vi "FieldByStepRotationForYakunin.vi"() -> ()   [LabVIEW 2019]
panel:
  in  "Rotator position Min":dbl
  in  "Rotator Position Max":dbl
  out "Direct Field Step:\nCurrent Value":dbl=0.1
  in  "Field Step Tab Control":enum32{"Direct Field", "Reciprocal Field"}(tab)
  in  "Direct Field Step (T)":dbl=0.1
  in  "DFS: Direct Field Step (T)":dbl=0.1
  in  "RFS: Reciprocal Field Step (1/T)":dbl=0.01
  in  "Threshold (T)":dbl=5.0
  in  "Calculate Setpoint":bool
  out "Power Supply State":string
  in  "Power Supply State":T1(ring)
  in  "Field:Rate [T/min]":dbl=0.2 min=0.0 max=0.6
  in  "Field:Final Setpoint":dbl min=-18.0 max=18.0
  out "Field: Current Value":dbl
  in  "stop":bool
  out "Field Runs":bool
  out "Field: Current Setpoint":dbl format="%.5f"
  out "Measurement Runs":bool
  in  "Steady Field":bool=TRUE
  # "Direct Field Step (DFS) will not be\nchanged below Threshold; while above: DFS=RFS*Field^2"
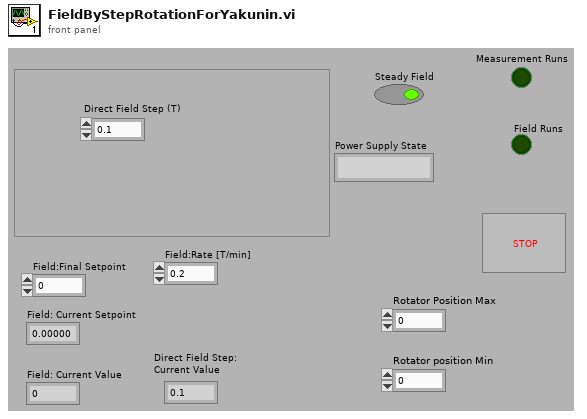
[diagram p1: front panel]
types:
  T1 = enum16{"No Response", "Ramping to programmed field ", "Holding at programmed field", "Paused", "Ramp Manual Up", "Ramp Manual Down", "Ramping to Zero", "QUENCH", "Heating Persistance Switch", "At Zero Current"}
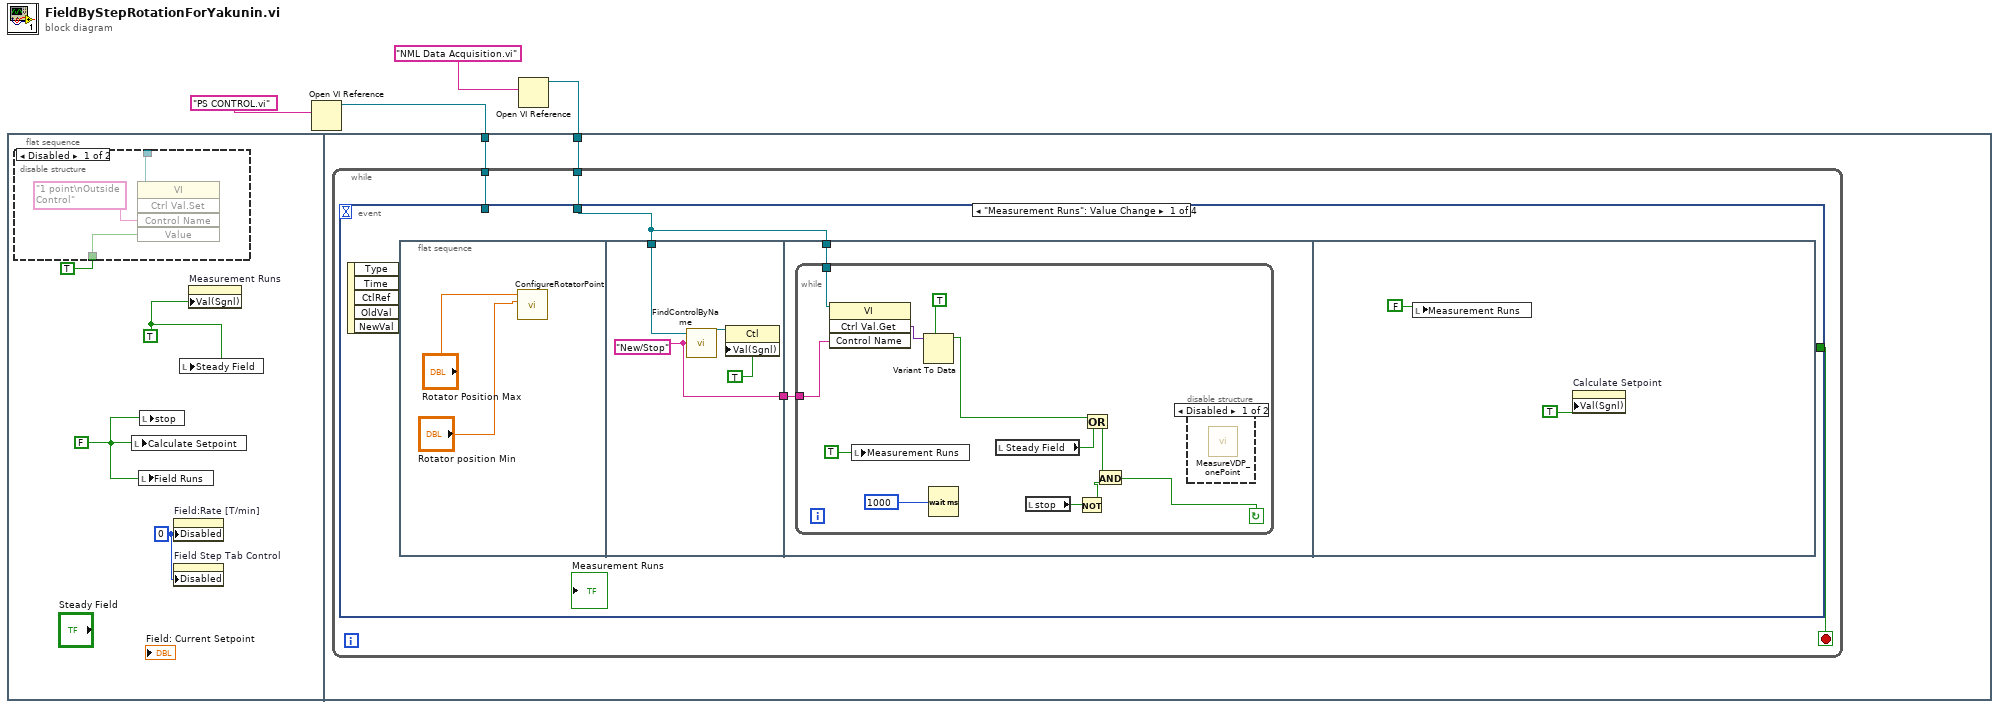
[diagram p0: block diagram]
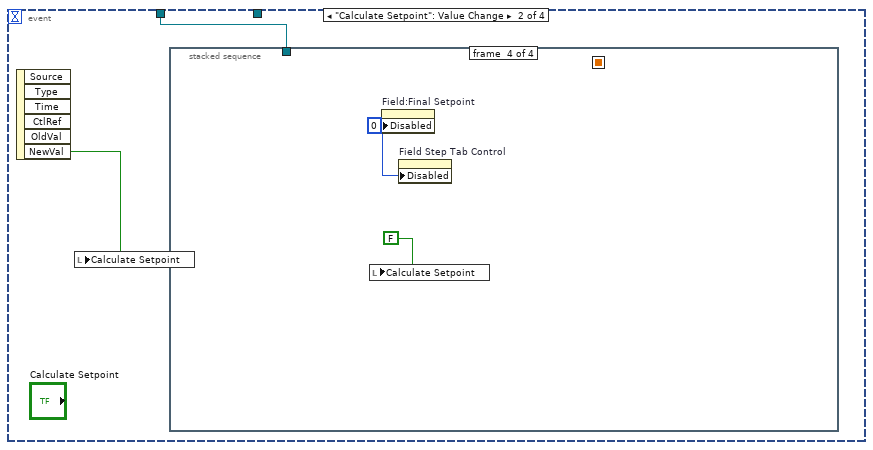
[diagram p4: hidden frame]
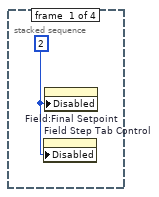
[diagram p5: hidden frame]
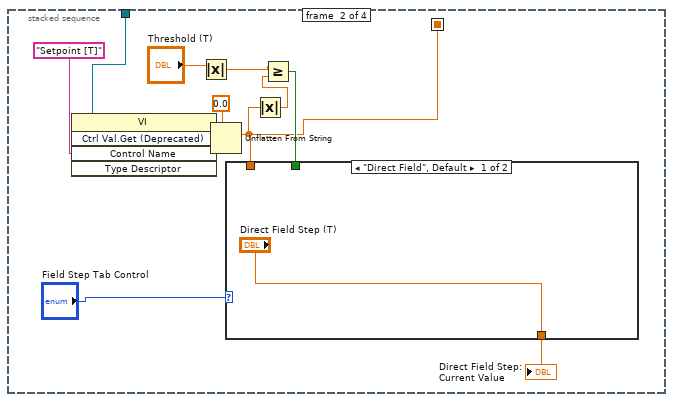
[diagram p6: hidden frame]
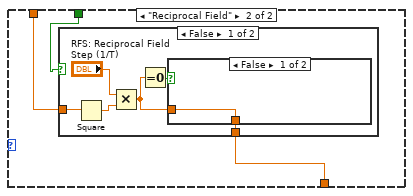
[diagram p7: hidden frame]
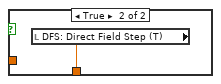
[diagram p8: hidden frame]
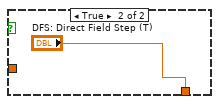
[diagram p9: hidden frame]
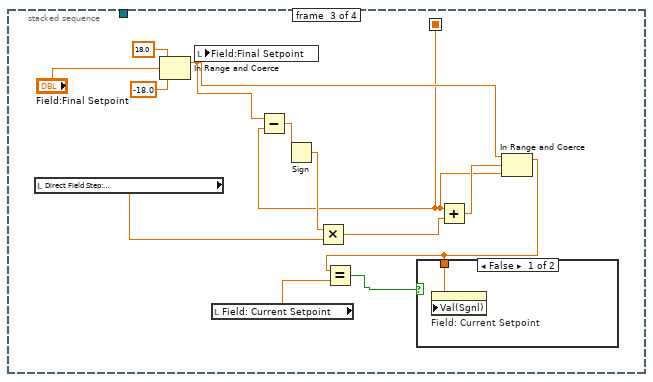
[diagram p10: hidden frame]
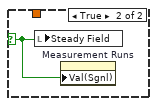
[diagram p11: hidden frame]
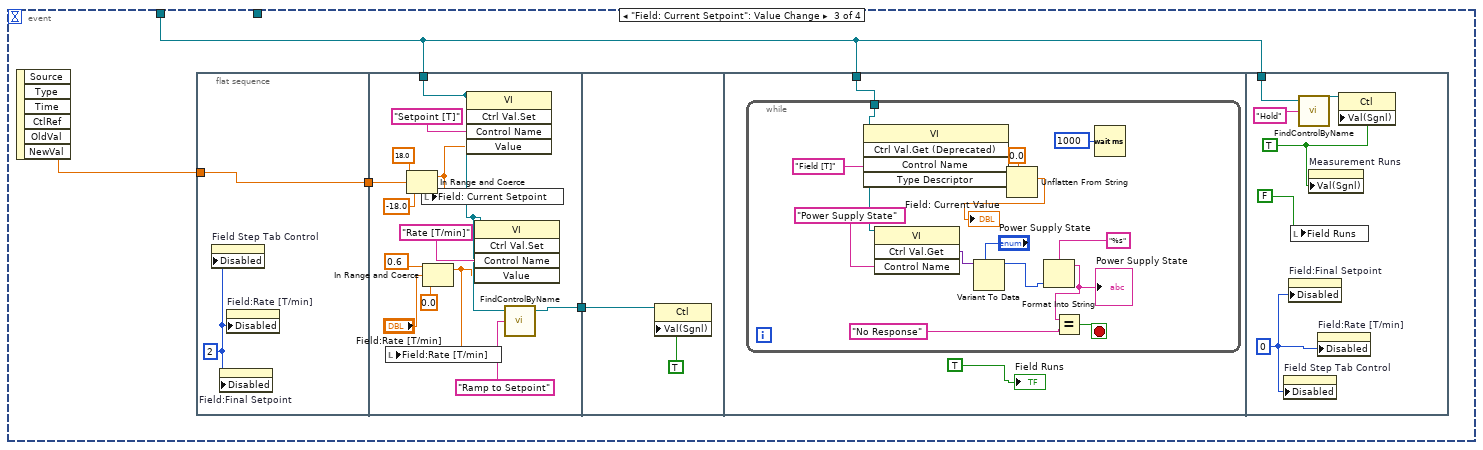
[diagram p12: hidden frame]
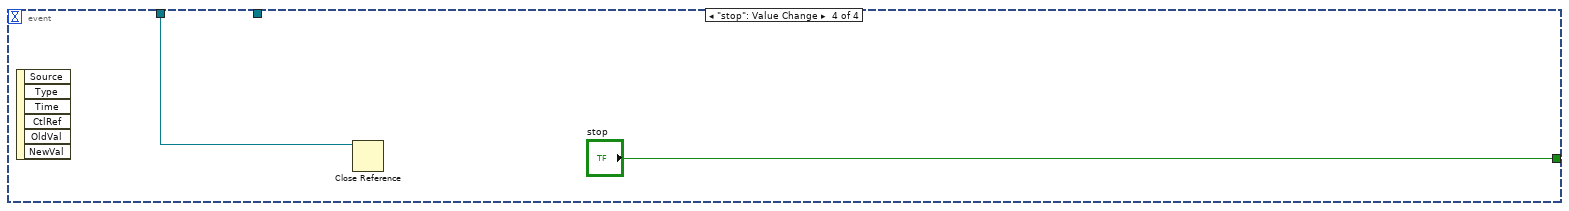
[diagram p13: hidden frame]
diagram:
  n1 = flat-sequence {
    tunnel: w3 -> [w13]
    tunnel: w1 -> [w12]
    frame #0 {
      w6 = u8 0 ("Disabled")
      w8 = FALSE ("Boolean")
      w7 = TRUE ("Boolean")
      n2 = disable-structure shown="Disabled" {
        disable-tunnel: TRUE ("Value (Signaling)") -> [w10 _]
        disable-tunnel: _ -> [w9 _]
        frame Disabled {
          n3 = invoke class="VI" method="Ctrl Val.Set"(reference=w9, "Control Name"="1 point\nOutside Control", "Value"=w10) -> ()  [unwired: 2 in, 5 out]
        }
        frame Enabled {
        }
      }
      n4 = local write "Calculate Setpoint"(w8) -> ()
      n5 = local write "Field Runs"(w8) -> ()
      n6 = local write "stop"(w8) -> ()
      n7 = property on="Field:Rate [T/min]" class="DigNum (strict)"("Disabled"=w6) -> ()  [unwired: 2 in, 2 out]
      n8 = property on="Field Step Tab Control" class="TabCtl (strict)"("Disabled"=w6) -> ()  [unwired: 2 in, 2 out]
      n9 = local write "Steady Field"(w7) -> ()
      n10 = property on="Measurement Runs" class="Bool (strict)"("Val(Sgnl)"=w7) -> ()  [unwired: 2 in, 2 out]
    }
    frame #1 {
      n11 = while {
        tunnel: w13 -> [w15]
        tunnel: w12 -> [w14]
        stop <- w16 stop-if-true
        n12 = event shown="[0] \"Measurement Runs\": Value Change" {
          selector: _ -> [_ _ _ _]
          dyn-events: _ -> [_ _ _ _]
          timeout: _ -> [_ _ _ _]
          tunnel: [_ _ _ "stop"] -> w16
          tunnel: w15 -> [_ w41 w87 w128]
          tunnel: w14 -> [w18 _ _ _]
          event "Measurement Runs": Value Change {
            n13 = event-data() -> ()  [unwired: 1 in, 5 out]
            n14 = flat-sequence {
              tunnel: w18 -> [w23]
              tunnel: [w21] -> w17
              tunnel: w18 -> [w26]
              tunnel: w17 -> [w25]
              frame #0 {
                n15 = call "ConfigureRotatorPoint.vi"("Rotator Position Min"="Rotator position Min", "Rotator Position Max"="Rotator Position Max") -> ()  [unwired: 10 in]
              }
              frame #1 {
                w21 = "New/Stop" ("Control Name")
                n16 = call "FindControlByName.vi"("control name"=w21, "vi refnum"=w23) -> ("control refnum"=w22:refnum<vi>)  [unwired: 2 in, 1 out]
                n17 = property class="Ctl"(reference=w22, "Val(Sgnl)"=TRUE ("Value (Signaling)")) -> ()  [unwired: 1 in, 2 out]
              }
              frame #2 {
                n18 = while {
                  tunnel: w26 -> [w33]
                  tunnel: w25 -> [w32]
                  stop <- w27 continue-if-true
                  n19 = invoke class="VI" method="Ctrl Val.Get"(reference=w33, "Control Name"=w32) -> ("Get Control Value Variant"=w34:variant)  [unwired: 2 in, 3 out]
                  n20 = local write "Measurement Runs"(TRUE ("Measurement Test")) -> ()
                  n21 = Variant To Data(type=TRUE ("Value (Signaling)"), Variant=w34) -> (data=w30:bool)  [unwired: 1 in, 1 out]
                  n22 = Wait (ms)(milliseconds to wait=u32 1000 ("millisecond timer value")) -> ()  [unwired: 1 out]
                  n23 = local read "Steady Field"() -> (w29:bool)
                  n24 = local read "stop"() -> (w36:bool)
                  n25 = Not(x=w36) -> (.not. x?=w35:bool)
                  n26 = Or(x=w30, y=w29) -> (x .or. y?=w28:bool)
                  n27 = And(x=w28, y=w35) -> (x .and. y?=w27:bool)
                  n28 = disable-structure shown="Disabled" {
                    frame Disabled {
                      n29 = call "MeasureVDP_onePoint.vi"() -> ()  [unwired: 1 in]
                    }
                    frame Enabled {
                    }
                  }
                }
              }
              frame #3 {
                n30 = local write "Measurement Runs"(FALSE ("Measurement Test")) -> ()
                n31 = property on="Calculate Setpoint" class="Bool (strict)"("Val(Sgnl)"=TRUE ("Value (Signaling)")) -> ()  [unwired: 2 in, 2 out]
              }
            }
          }
          event "Calculate Setpoint": Value Change {
            n32 = event-data() -> ("NewVal"=w42:bool)  [unwired: 1 in, 5 out]
            n33 = local write "Calculate Setpoint"(w42) -> ()
            n34 = stacked-sequence {
              seq-local: [_ w45 _ _] -> [_ _ w69 _]
              tunnel: w41 -> [_ w50 _ _]
              frame #0 {
                w43 = u8 2 ("Disabled")
                n35 = property on="Field Step Tab Control" class="TabCtl (strict)"("Disabled"=w43) -> ()  [unwired: 2 in, 2 out]
                n36 = property on="Field:Final Setpoint" class="DigNum (strict)"("Disabled"=w43) -> ()  [unwired: 2 in, 2 out]
              }
              frame #1 {
                n37 = invoke class="VI" method="Ctrl Val.Get (Deprecated)"(reference=w50, "Control Name"="Setpoint [T]") -> ("Get Control Value"=w52:string)  [unwired: 3 in, 4 out]
                n38 = Absolute Value(x="Threshold (T)") -> (abs(x)=w47:dbl)
                n39 = Unflatten From String(type=0.0, binary string=w52) -> (value=w45:dbl)  [unwired: 3 in, 2 out]
                n40 = Absolute Value(x=w45) -> (abs(x)=w48:dbl)
                n41 = Greater Or Equal?(x=w47, y=w48) -> (x >= y?=w46:bool)
                n42 = case shown="\"Direct Field\", Default" "Field Step Tab Control" {
                  tunnel: w46 -> [_ w58]
                  tunnel: w45 -> [_ w57]
                  tunnel: ["Direct Field Step (T)" w56] -> w44
                  frame "Direct Field", Default {
                  }
                  frame "Reciprocal Field" {
                    n43 = case shown="False" w58 {
                      tunnel: w57 -> [w62 _]
                      tunnel: [w59 "DFS: Direct Field Step (T)"] -> w56
                      frame False {
                        n44 = Square(x=w62) -> (x^2=w63:dbl)
                        n45 = Multiply(x="RFS: Reciprocal Field Step (1/T)", y=w63) -> (x*y=w60:dbl)
                        n46 = Equal To 0?(x=w60) -> (x = 0?=w61:bool)
                        n47 = case shown="False" w61 {
                          tunnel: w60 -> [w65 _]
                          tunnel: [w65 w66] -> w59
                          frame False {
                          }
                          frame True {
                            n48 = local read "DFS: Direct Field Step (T)"() -> (w66:dbl)
                          }
                        }
                      }
                      frame True {
                      }
                    }
                  }
                }
                "Direct Field Step:\nCurrent Value" <- w44
              }
              frame #2 {
                n49 = local read "Direct Field Step:\nCurrent Value"() -> (w68:dbl)
                n50 = In Range and Coerce(upper limit=18.0, x="Field:Final Setpoint", lower limit=-18.0) -> (coerced(x)=w70:dbl)  [unwired: 1 out]
                n51 = local write "Field:Final Setpoint"(w70) -> ()
                n52 = local read "Field: Current Setpoint"() -> (w74:dbl)
                n53 = Subtract(x=w70, y=w69) -> (x-y=w78:dbl)
                n54 = Sign(1:w78) -> (0:w77:dbl)
                n55 = Multiply(x=w77, y=w68) -> (x*y=w76:dbl)
                n56 = Add(x=w69, y=w76) -> (x+y=w75:dbl)
                n57 = In Range and Coerce(upper limit=w70, x=w75, lower limit=w69) -> (coerced(x)=w72:dbl)  [unwired: 1 out]
                n58 = Equal?(x=w72, y=w74) -> (x = y?=w73:bool)
                n59 = case shown="False" w73 {
                  selector: w73 -> [_ w82]
                  tunnel: w72 -> [w81 _]
                  frame False {
                    n60 = property on="Field: Current Setpoint" class="DigNum (strict)"("Val(Sgnl)"=w81) -> ()  [unwired: 2 in, 2 out]
                  }
                  frame True {
                    n61 = local write "Steady Field"(w82) -> ()
                    n62 = property on="Measurement Runs" class="Bool (strict)"("Val(Sgnl)"=w82) -> ()  [unwired: 2 in, 2 out]
                  }
                }
              }
              frame #3 {
                w83 = u8 0 ("Disabled")
                n63 = local write "Calculate Setpoint"(FALSE ("Calculate Setpoint")) -> ()
                n64 = property on="Field:Final Setpoint" class="DigNum (strict)"("Disabled"=w83) -> ()  [unwired: 2 in, 2 out]
                n65 = property on="Field Step Tab Control" class="TabCtl (strict)"("Disabled"=w83) -> ()  [unwired: 2 in, 2 out]
              }
            }
          }
          event "Field: Current Setpoint": Value Change {
            n66 = event-data() -> ("NewVal"=w88:dbl)  [unwired: 1 in, 5 out]
            n67 = flat-sequence {
              tunnel: w88 -> [w90]
              tunnel: [w90] -> w85
              tunnel: w87 -> [w97]
              tunnel: [w99] -> w86
              tunnel: w85 -> [w101]
              tunnel: w86 -> [w105]
              tunnel: w87 -> [w107]
              tunnel: w87 -> [w125]
              frame #0 {
                w89 = u8 2 ("Disabled")
                n68 = property on="Field Step Tab Control" class="TabCtl (strict)"("Disabled"=w89) -> ()  [unwired: 2 in, 2 out]
                n69 = property on="Field:Final Setpoint" class="DigNum (strict)"("Disabled"=w89) -> ()  [unwired: 2 in, 2 out]
                n70 = property on="Field:Rate [T/min]" class="DigNum (strict)"("Disabled"=w89) -> ()  [unwired: 2 in, 2 out]
              }
              frame #1 {
                n71 = In Range and Coerce(upper limit=18.0, x=w101, lower limit=-18.0) -> (coerced(x)=w91:dbl)  [unwired: 1 out]
                n72 = local write "Field: Current Setpoint"(w91) -> ()
                n73 = In Range and Coerce(upper limit=0.6 ("x"), x="Field:Rate [T/min]", lower limit=0.0) -> (coerced(x)=w93:dbl)  [unwired: 1 out]
                n74 = local write "Field:Rate [T/min]"(w93) -> ()
                n75 = invoke class="VI" method="Ctrl Val.Set"(reference=w97, "Control Name"="Setpoint [T]", "Value"=w91) -> ()  [unwired: 2 in, 5 out]
                n76 = invoke class="VI" method="Ctrl Val.Set"(reference=w97, "Control Name"="Rate [T/min]", "Value"=w93) -> ()  [unwired: 2 in, 5 out]
                n77 = call "FindControlByName.vi"("control name"="Ramp to Setpoint" ("Control Name"), "vi refnum"=w97) -> ("control refnum"=w99:refnum<vi>)  [unwired: 2 in, 1 out]
              }
              frame #2 {
                n78 = property class="Ctl"(reference=w105, "Val(Sgnl)"=TRUE ("Value (Signaling)")) -> ()  [unwired: 1 in, 2 out]
              }
              frame #3 {
                n79 = while {
                  tunnel: w107 -> [w118]
                  stop <- w121 stop-if-true
                  n80 = invoke class="VI" method="Ctrl Val.Get (Deprecated)"(reference=w118, "Control Name"="Field [T]") -> ("Get Control Value"=w120:string)  [unwired: 3 in, 4 out]
                  n81 = invoke class="VI" method="Ctrl Val.Get"(reference=w118, "Control Name"="Power Supply State") -> ("Get Control Value Variant"=w114:variant)  [unwired: 2 in, 3 out]
                  n82 = Variant To Data(type="Power Supply State", Variant=w114) -> (data=w110:T1)  [unwired: 1 in, 1 out]
                  n83 = Unflatten From String(type=0.0, binary string=w120) -> (value=→"Field: Current Value":dbl)  [unwired: 3 in, 2 out]
                  n84 = Format Into String(format string="%s", w110) -> (resulting string=w112:string)  [unwired: 2 in, 1 out]
                  "Power Supply State" <- w112
                  n85 = Equal?(x=w112, y="No Response") -> (x = y?=w121:bool)
                  n86 = Wait (ms)(milliseconds to wait=u32 1000 ("millisecond timer value")) -> ()  [unwired: 1 out]
                }
                "Field Runs" <- TRUE ("Field Test")
              }
              frame #4 {
                w122 = u8 0 ("Disabled")
                w123 = TRUE ("Value (Signaling)")
                n87 = property on="Field Step Tab Control" class="TabCtl (strict)"("Disabled"=w122) -> ()  [unwired: 2 in, 2 out]
                n88 = property on="Field:Final Setpoint" class="DigNum (strict)"("Disabled"=w122) -> ()  [unwired: 2 in, 2 out]
                n89 = local write "Field Runs"(FALSE ("Field Test")) -> ()
                n90 = call "FindControlByName.vi"("control name"="Hold" ("Control Name"), "vi refnum"=w125) -> ("control refnum"=w126:refnum<vi>)  [unwired: 2 in, 1 out]
                n91 = property on="Measurement Runs" class="Bool (strict)"("Val(Sgnl)"=w123) -> ()  [unwired: 2 in, 2 out]
                n92 = property on="Field:Rate [T/min]" class="DigNum (strict)"("Disabled"=w122) -> ()  [unwired: 2 in, 2 out]
                n93 = property class="Ctl"(reference=w126, "Val(Sgnl)"=w123) -> ()  [unwired: 1 in, 2 out]
              }
            }
          }
          event "stop": Value Change {
            n94 = event-data() -> ()  [unwired: 1 in, 6 out]
            n95 = Close Reference(reference=w128) -> ()  [unwired: 1 in, 1 out]
          }
        }
      }
    }
  }
  n96 = Open VI Reference(vi path="PS CONTROL.vi") -> (vi reference=w3:refnum<vi>)  [unwired: 5 in, 1 out]
  n97 = Open VI Reference(vi path="NML Data Acquisition.vi") -> (vi reference=w1:refnum<vi>)  [unwired: 5 in, 1 out]
